vi "Log.vi"(7 "Source":string, 8 "error in (no error)":errorcluster, 9 "Message":string, 10 "Level":T1, 11 "Log Indicator In":refnum<class "Log Indicator.lvclass">) -> (0 "error out":errorcluster, 3 "Log Indicator Out":refnum<class "Log Indicator.lvclass">)   [LabVIEW 2020, in "Log Indicator.lvclass"]
doc: "Enter a message into the system log."
uses:
  <vilib>/Asteme/Triarc Framework/Logging/Protected/Level.ctl
  Log Indicator.lvclass
  <vilib>/Asteme/Triarc Framework/Logging/Logging.lvclass
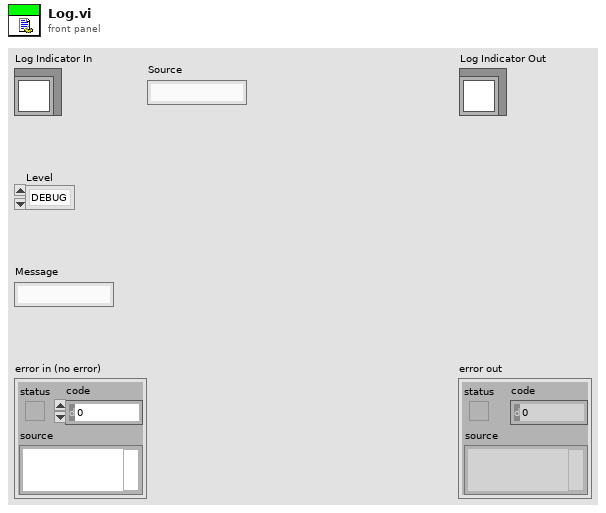
[diagram p1: front panel]
types:
  T1 = typedef "TF.lvlib/Logging.lvclass/Level.ctl" = enum16{"DEBUG", "INFO", "WARNING", "ERROR", "CRITICAL"}
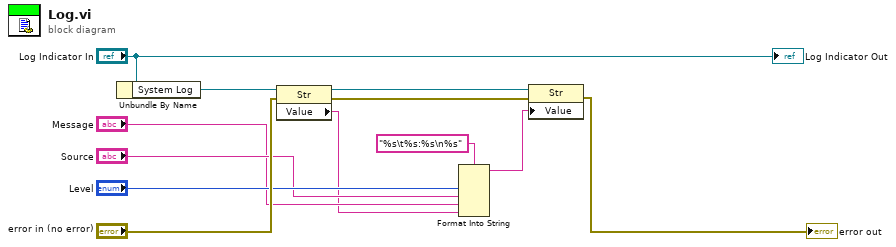
[diagram p0: block diagram]
diagram:
  n1 = Unbundle By Name("Log Indicator In") -> ("System Log"=w11:refnum<vi>)
  n2 = property class="Str"(reference=w11, error in="error in (no error)") -> (reference out=w10:refnum<vi>, error out=w9:errorcluster, "Value"=w2:string)
  n3 = Format Into String(format string="%s\t%s:%s\n%s", "Level", "Source", "Message", w2) -> (resulting string=w1:string)  [unwired: 2 in, 1 out]
  n4 = property class="Str"(reference=w10, error in=w9, "Value"=w1) -> (error out=→"error out":errorcluster)  [unwired: 1 out]
  "Log Indicator Out" <- "Log Indicator In"
